vi "calc.vi"(5 "Input Current":dbl[](array[numeric]), 6 "Input voltage":dbl[](array[numeric]), 7 "Area factor":dbl=1.0) -> (0 "Current":dbl format="%#.3f", 1 "Voltage":dbl format="%#.3f", 2 "Energy":dbl format="%#.3f", 3 "Power":dbl format="%#.3f", 4 "Waveform Chart":dynamicdata(graph))   [LabVIEW 2012]
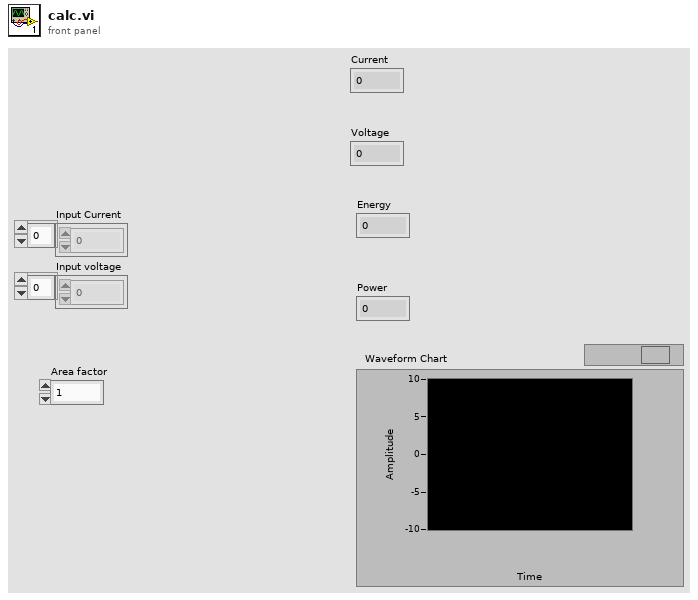
[diagram p1: front panel]
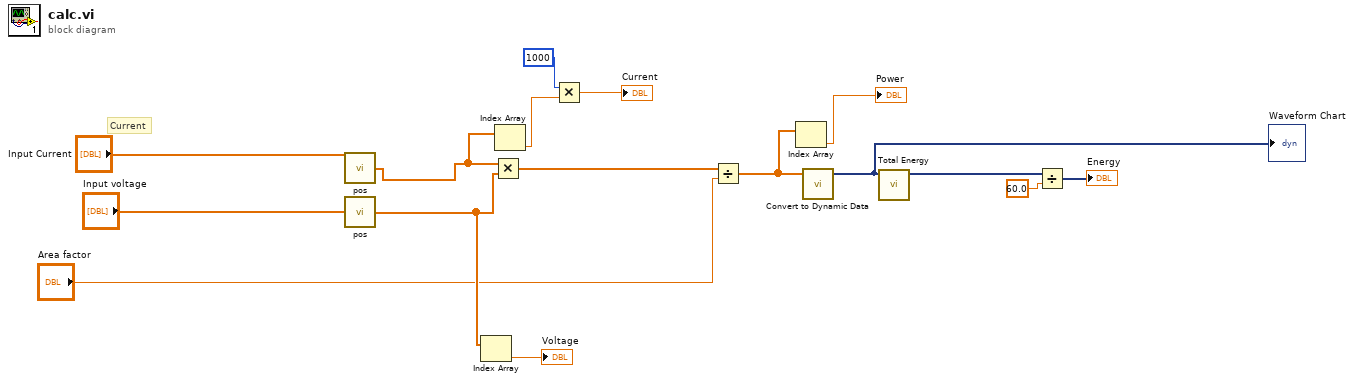
[diagram p0: block diagram]
diagram:
  # "Current"
  n1 = call "pos.vi"("Input"="Input Current") -> ("Output"=w3:dbl[])
  n2 = call "pos.vi"("Input"="Input voltage") -> ("Output"=w6:dbl[])
  n3 = Index Array(array=w6) -> (element=→"Voltage":dbl)  [unwired: 1 in]
  n4 = Multiply(x=w3, y=w6) -> (x*y=w13:dbl[])
  n5 = Index Array(array=w3) -> (element=w2:dbl)  [unwired: 1 in]
  n6 = Multiply(x=1000, y=w2) -> (x*y=→"Current":dbl)
  n7 = Divide(x=w13, y="Area factor") -> (x/y=w12:dbl[])
  n8 = Index Array(array=w12) -> (element=→"Power":dbl)  [unwired: 1 in]
  n9 = call "Convert to Dynamic Data"("Array"=w12) -> ("Dynamic Data Type"=w4:dynamicdata)  [unwired: 3 in]
  "Waveform Chart" <- w4
  n10 = call "Total Energy"("Signals"=w4) -> ("Result"=w15:dynamicdata)  [unwired: 5 in, 1 out]
  n11 = Divide(x=w15, y=60.0) -> (x/y=→"Energy":dynamicdata)
